vi "Lanuch New Chat Window.vi"(8 "error in (no error)":errorcluster, 11 "Server in":refnum<class "Server.lvclass">) -> (0 "error out":errorcluster, 3 "Server out":refnum<class "Server.lvclass">)   [LabVIEW 2020, in "Server.lvlib" / "Server.lvclass"]
uses:
  Server.lvclass
  C:/Program Files (x86)/National Instruments/LabVIEW 2020/vi.lib/ActorFramework/Actor/Actor.lvclass
  Chat Room Model/Chat Room Model/Chat Room Model.lvclass
  UI Status Update/User Info.ctl
  Chat Room Model/Chat Room Model/Chat Room Model.lvclass/Chat Room Model.ctl
  Server.lvclass/Server.ctl
  <vilib>/ActorFramework/Actor/Actor.lvclass/Actor.ctl
  <vilib>/ActorFramework/Message Enqueuer/Message Enqueuer.lvclass/Message Enqueuer.ctl
  Chat Room Model/Chat Room Model Messages/Update Online List Msg/Update Online List Msg.lvclass/Update Online List Msg.ctl
  Chat Room Model/Chat Room Model Messages/Update Online Status List Msg/Update Online Status List Msg.lvclass/Update Online Status List Msg.ctl
  Server Messages/Enable Controls Msg/Enable Controls Msg.lvclass/Enable Controls Msg.ctl
  <vilib>/ActorFramework/Message Enqueuer/Enqueue.vi
  <vilib>/ActorFramework/Message Enqueuer/Init from Existing Queue.vi
  Chat Room Model/Chat Room Model Messages/Update Online List Msg/Update Online List Msg.lvclass
  C:/Program Files (x86)/National Instruments/LabVIEW 2020/vi.lib/ActorFramework/Message/Message.lvclass
  Chat Room Model/Chat Room Model Messages/Update Online Status List Msg/Update Online Status List Msg.lvclass
  Server Messages/Enable Controls Msg/Enable Controls Msg.lvclass
  <vilib>/ActorFramework/Message Priority Queue/Priority Enqueue.vi
  <vilib>/ActorFramework/Message Enqueuer/Message Enqueuer.lvclass
  <vilib>/ActorFramework/Actor/Actor.lvclass
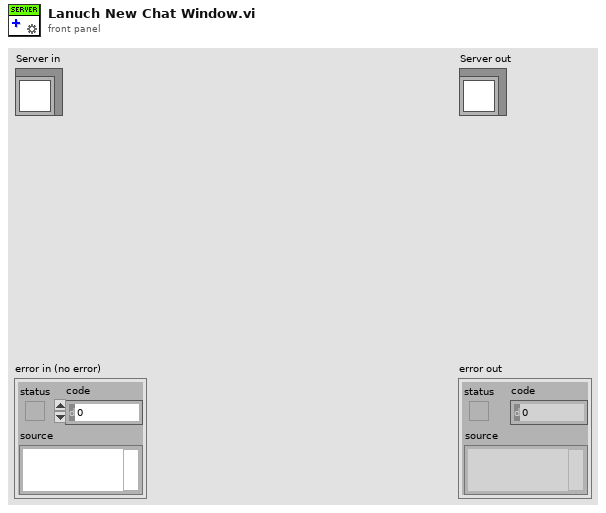
[diagram p1: front panel]
types:
  T1 = enum8{"Enabled", "Disabled", "Disabled and Grayed Out"}
  T2 = typedef "Chat Room Model.lvlib/Chat Room Model.lvclass/User Info.ctl" = cluster{"Name":string, "Status":string}
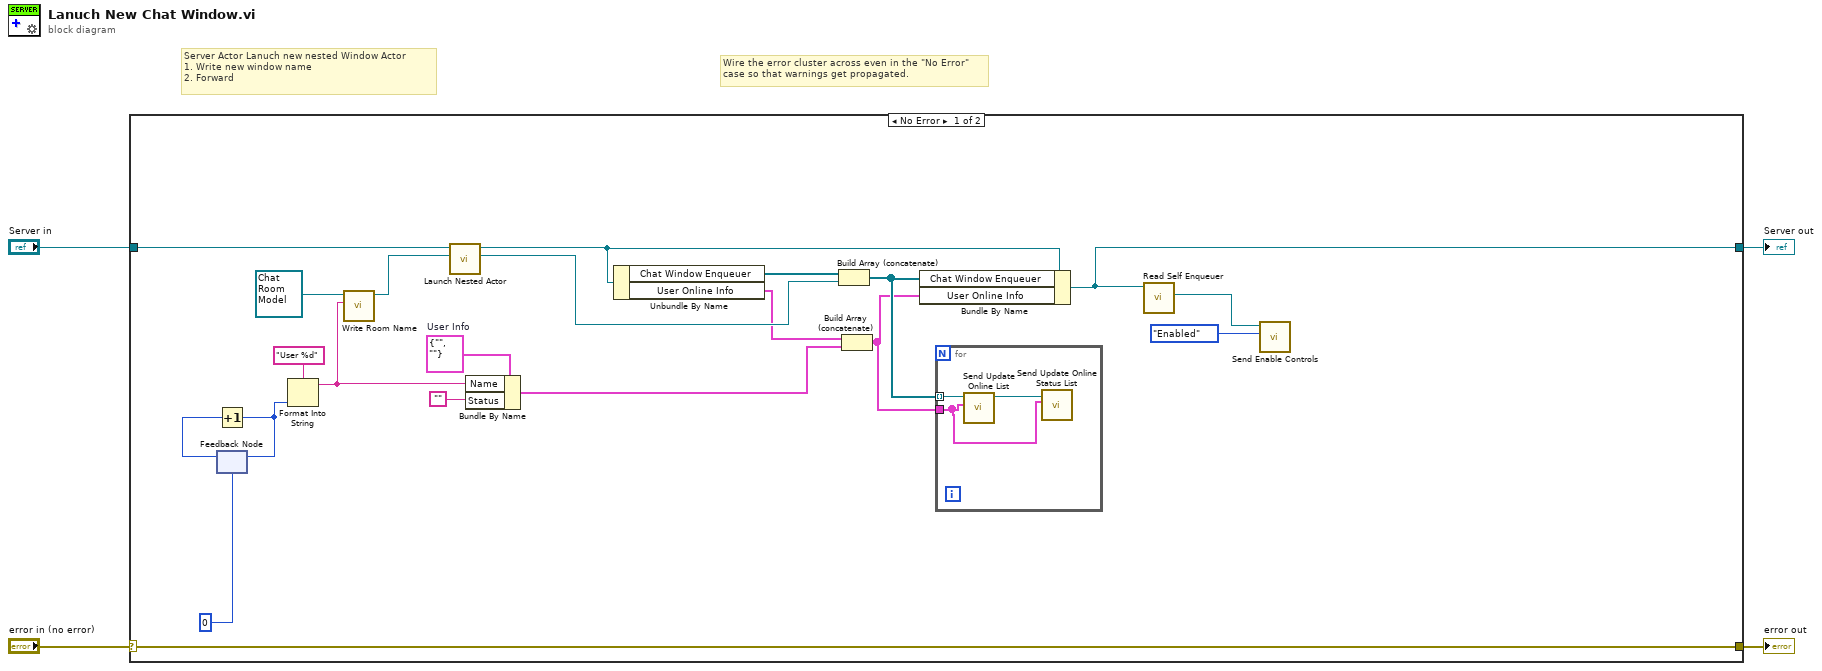
[diagram p0: block diagram]
diagram:
  # "Wire the error cluster across even in the \"No Error\"\ncase so that warnings get propagated."
  # "Server Actor Lanuch new nested Window Actor \n1. Write new window name\n2. Forward"
  n1 = case shown="No Error" "error in (no error)" {
    selector: "error in (no error)" -> [w25 w30]
    tunnel: [w25 w30] -> w3
    tunnel: [w9 w29] -> w1
    tunnel: "Server in" -> [w24 w29]
    frame No Error {
      w14 = T2 {"Name"="", "Status"=""}  # User Info
      n2 = feedback #1(0) -> (w17:i32)
      n3 = Increment(x=w17) -> (x+1=w15:i32)
      n4 = feedback-in #1(w15) -> ()
      n5 = Format Into String(format string="User %d", w15) -> (resulting string=w10:string)  [unwired: 2 in, 1 out]
      n6 = call "Write Room Name.vi"("Room Name"=w10, "Chat Room Model in"=refnum<class "Chat Room Model.lvclass"> refnum ("Chat Room Model.lvlib:Chat Room Model.lvclass")) -> ("Chat Room Model out"=w19:refnum<class "Chat Room Model.lvclass">)  [unwired: 8 in, 1 out]
      n7 = call <vilib>:"Launch Nested Actor.vi"("Nested Actor"=w19, "Caller Actor in"=w24) -> ("Nested Actor's Enqueuer"=w22:refnum<class "Message Enqueuer.lvclass">, "Caller Actor out"=w21:refnum<class "Server.lvclass">)  [unwired: 7 in, 1 out]
      n8 = Bundle By Name(cluster=w14, "Name"=w10, "Status"="") -> (w13:T2)
      n9 = Unbundle By Name(w21) -> ("Chat Window Enqueuer"=w23:refnum<class "Message Enqueuer.lvclass">[], "User Online Info"=w12:T2[])
      n10 = Build Array (concatenate)(w23, w22) -> (w11:refnum<class "Message Enqueuer.lvclass">[])
      n11 = Build Array (concatenate)(w12, w13) -> (w5:T2[])
      n12 = Bundle By Name(cluster=w21, "Chat Window Enqueuer"=w11, "User Online Info"=w5) -> (w9:refnum<class "Server.lvclass">)
      n13 = for {
        tunnel: w11 -> [w28] mode=indexing
        tunnel: w5 -> [w26]
        n14 = call "Send Update Online List.vi"("User Online Info"=w26, "Message Enqueuer"=w28) -> ("Message Enqueuer out"=w27:refnum<class "Message Enqueuer.lvclass">)  [unwired: 8 in, 1 out]
        n15 = call "Send Update Online Status List.vi"("User Online Info"=w26, "Message Enqueuer"=w27) -> ()  [unwired: 8 in, 2 out]
      }
      n16 = call <vilib>:"Read Self Enqueuer.vi"("Actor"=w9) -> ("Self Enqueuer"=w8:refnum<class "Message Enqueuer.lvclass">)  [unwired: 10 in]
      n17 = call "Send Enable Controls.vi"("Disabled"=T1."Enabled", "Message Enqueuer"=w8) -> ()  [unwired: 8 in, 2 out]
    }
    frame Error {
    }
  }
  "error out" <- w3
  "Server out" <- w1
